vi "Setup for Get File Content.vi"(8 "error in":errorcluster, 11 "File Name":string="file.txt") -> (0 "error out":errorcluster, 3 "read file.lvclass":refnum<class "Read File.lvclass">)   [LabVIEW 2023]
doc: "This VI calls the Write File Refnum VI to pass the file name to Read File.lvclass. Use this VI as a setup VI for the Get File Content.lvtest test."
uses:
  Read File.lvclass
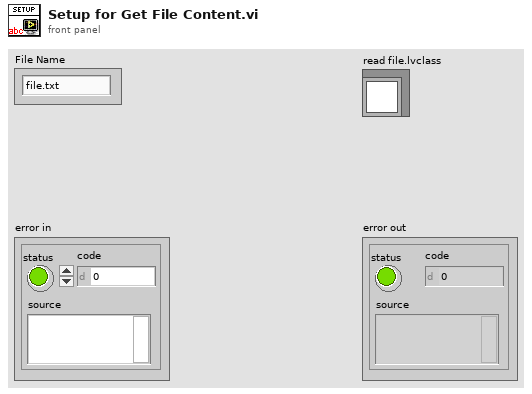
[diagram p1: front panel]
types:
  T1 = enum16{"open", "replace", "create", "open or create", "replace or create", "replace or create with confirmation"}
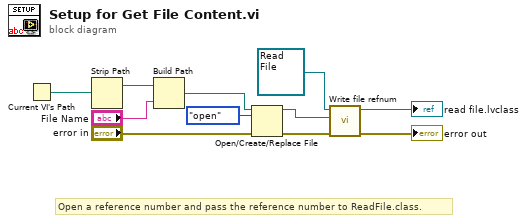
[diagram p0: block diagram]
diagram:
  # "Open a reference number and pass the reference number to ReadFile.class."
  n1 = Current VI's Path() -> (path=w6:path)
  n2 = Strip Path(path=w6) -> (stripped path=w5:path)  [unwired: 1 out]
  n3 = Build Path(base path=w5, name or relative path="File Name") -> (appended path=w3:path)
  n4 = Open/Create/Replace File(file path (use dialog)=w3, error in="error in", operation (0:open)=T1."open") -> (refnum out=w8:refnum<file>, error out=w9:errorcluster)  [unwired: 3 in, 1 out]
  n5 = call "Write file refnum.vi"("error in (no error)"=w9, "file refnum"=w8, "read file in"=refnum<class "Read File.lvclass"> refnum) -> ("error out"=→"error out":errorcluster, "read file out"=→"read file.lvclass":refnum<class "Read File.lvclass">)  [unwired: 7 in]
